vi "Factory Create.vi"(8 "Error In":errorcluster, 10 "IConfigure":refnum<class "IConfigure.lvclass">, 11 "reference in":refnum<class "Voltmeter Virtual.lvclass">) -> (0 "Error Out":errorcluster, 3 "reference out":refnum<class "Voltmeter Virtual.lvclass">)   [LabVIEW 2023, in "Voltmeter Virtual.lvlib" / "Voltmeter Virtual.lvclass"]
uses:
  Voltmeter Virtual.lvclass
  Interfaces/IConfigure/IConfigure.lvclass
  Voltmeter Virtual.lvclass/Voltmeter Virtual.ctl
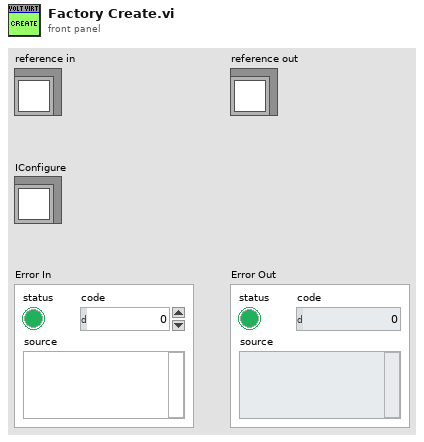
[diagram p1: front panel]
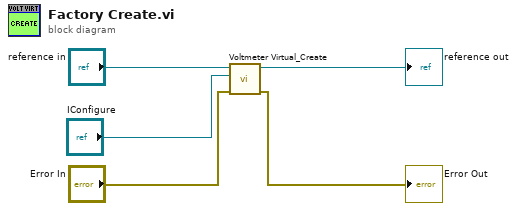
[diagram p0: block diagram]
diagram:
  n1 = call "Voltmeter Virtual_Create.vi"("Error In"="Error In", "IConfigure"="IConfigure", "reference in"="reference in") -> ("Error Out"=→"Error Out":errorcluster, "reference out"=→"reference out":refnum<class "Voltmeter Virtual.lvclass">)  [unwired: 7 in]
